vi "Build Return to High Priority Check.vi"(7 "Virtual Memory Unit in":refnum<class "Virtual Memory Unit.lvclass">, 8 "error in (no error)":errorcluster, 10 "Starting Address":u16 format="%04x", 11 "Major Frame in":refnum<class "Major Frame.lvclass">) -> (0 "error out":errorcluster, 2 "Next Available Address":u16 format="%04x", 3 "Major Frame out":refnum<class "Major Frame.lvclass">, 5 "Virtual Memory Unit out":refnum<class "Virtual Memory Unit.lvclass">)   [LabVIEW 2016, in "BCI-1553 API.lvlib" / "Major Frame.lvclass"]
doc: "Checks if there's enough time to watch for high or low priority message requests. If not, the sequence advances as normal. If there is time, the sequence execution returns to the group 0 high priority check."
uses:
  Major Frame.lvclass
  TypeDefs/BC Condition Codes.ctl
  BCI-1553 API.lvlib
  TypeDefs/BC Op Codes - Verbose.ctl
  Dependencies/Virtual Memory Unit/Virtual Memory Unit.lvclass
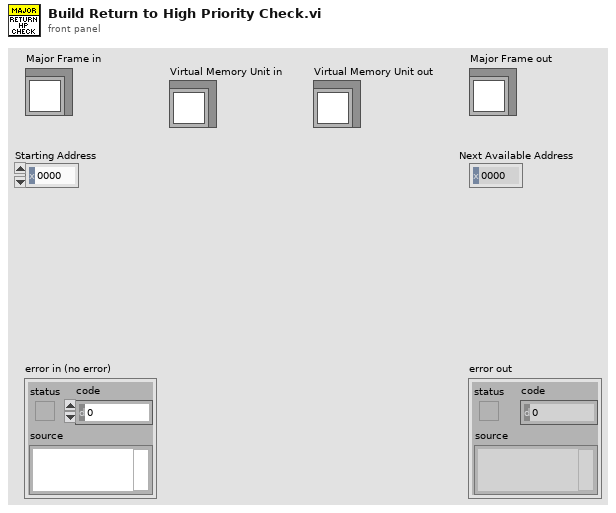
[diagram p1: front panel]
types:
  T1 = typedef "BCI-1553 API.lvlib/BC Op Codes - Verbose.ctl" = enum16{"EXECUTE MSG", "EXECUTE MSG GO", "JUMP", "CALL SUBROUTINE", "RETURN", "INTERRUPT REQUEST", "HALT", "DELAY", "WAIT FRAME TIMER = 0", "COMPARE FRAME TIMER", "COMPARE MSG TIMER", "LOAD TIME TAG CTR", "LOAD TIME TAG CTR HI", "LOAD FRAME TIMER", "START FRAME TIMER", "PUSH TIME TAG COUNT", "PUSH TIME TAG COUNT HI", "PUSH TIME TAG COUNT BOTH", "PUSH BLOCK STATUS WORD", "PUSH CURRENT VALUE", "PUSH INDIRECT", "WAIT EXT TRIGGER", "EXECUTE AND FLIP", "EXECUTE, FLIP, GO", "WRITE VALUE TO WMI", "WRITE VALUE TO MEM", "DECREMENT RAM, SKIP", "FLAG"}
  T2 = typedef "BCI-1553 API.lvlib/BC Condition Codes.ctl" = enum16{"GP0 == 1 || LT", "GP1 == 1 || NE", "GP2 == 1", "GP3 == 1", "GP4 == 1", "GP5 == 1", "GP6 == 1", "GP7 == 1", "NORESP", "FMTERR", "GOODBLOCK", "MSKSTATSET", "BADMSG", "1RETRY", "2RETRY", "ALWAYS"}
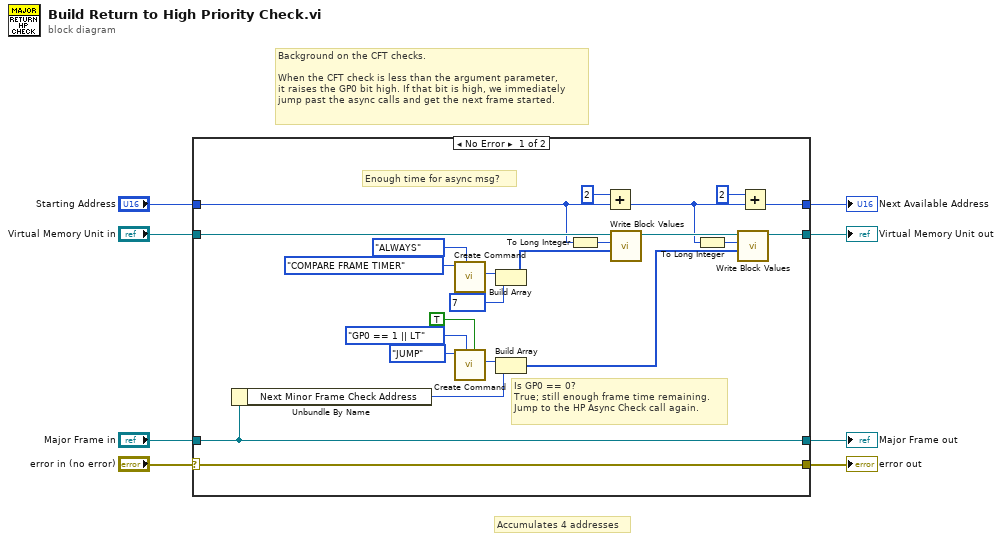
[diagram p0: block diagram]
diagram:
  # "Background on the CFT checks.\n\nWhen the CFT check is less than the argument parameter,\nit raises the GP0 bit high. If that bit is high, we immediately\njump past the async calls and get the next frame started."
  # "Accumulates 4 addresses"
  n1 = case shown="No Error" "error in (no error)" {
    selector: "error in (no error)" -> [w31 w35]
    tunnel: [w31 w35] -> w7
    tunnel: [w10 w34] -> w5
    tunnel: "Major Frame in" -> [w10 w34]
    tunnel: "Virtual Memory Unit in" -> [w14 w32]
    tunnel: "Starting Address" -> [w13 w33]
    tunnel: [w12 w33] -> w2
    tunnel: [w11 w32] -> w1
    frame No Error {
      # "Is GP0 == 0?\nTrue; still enough frame time remaining.\nJump to the HP Async Check call again."
      # "Enough time for async msg?"
      n2 = Unbundle By Name(w10) -> ("Next Minor Frame Check Address"=w9:u16)
      n3 = call "Create Command.vi"("Condition"=BC_Condition_Codes."ALWAYS", "Op Code"=BC_Op_Codes_-_Verbose."COMPARE FRAME TIMER") -> ("Instruction"=w28:u16)  [unwired: 8 in, 1 out]
      n4 = call "Create Command.vi"("Invert Condition (F)"=TRUE, "Condition"=BC_Condition_Codes."GP0 == 1 || LT", "Op Code"=BC_Op_Codes_-_Verbose."JUMP") -> ("Instruction"=w22:u16)  [unwired: 7 in, 1 out]
      n5 = Build Array(w28, u16 7 ("element")) -> (w26:u16[])
      n6 = Build Array(w22, w9) -> (w23:u16[])
      n7 = To Long Integer(number=w13) -> (32bit integer=w25:i32)
      n8 = Add(x=u16 2, y=w13) -> (x+y=w18:u16)
      n9 = call "Write Block Values.vi"("Write Block"=w26, "Start Index"=w25, "Virtual Memory Unit in"=w14) -> ("Virtual Memory Unit out"=w19:refnum<class "Virtual Memory Unit.lvclass">)  [unwired: 7 in, 1 out]
      n10 = To Long Integer(number=w18) -> (32bit integer=w24:i32)
      n11 = call "Write Block Values.vi"("Write Block"=w23, "Start Index"=w24, "Virtual Memory Unit in"=w19) -> ("Virtual Memory Unit out"=w11:refnum<class "Virtual Memory Unit.lvclass">)  [unwired: 7 in, 1 out]
      n12 = Add(x=u16 2, y=w18) -> (x+y=w12:u16)
    }
    frame Error {
    }
  }
  "error out" <- w7
  "Major Frame out" <- w5
  "Next Available Address" <- w2
  "Virtual Memory Unit out" <- w1
